vi "Cron Time to TimeStamp.vi"(10 "Correct for DST?":bool, 11 "Cron Time":T1) -> (3 "Time Stamp":timestamp)   [LabVIEW 2013, in "openCron.lvlib" / "Cron.lvclass"]
uses:
  Cron.lvclass
  CronTime -- cluster.ctl
  <vilib>/Utility/miscctls.llb/LVDateTimeRec.ctl
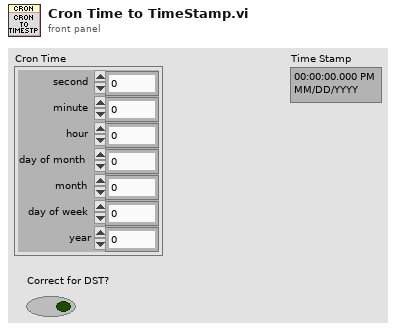
[diagram p1: front panel]
types:
  T1 = typedef "openCron.lvlib/Cron.lvclass/CronTime -- cluster.ctl" = cluster{"second":i32, "minute":i32, "hour":i32, "day of month":i32, "month":i32, "day of week":i32, "year":i32}
  T2 = typedef "LVDateTimeRec.ctl" = cluster{"fractional second":dbl, "second":i32, "minute":i32, "hour":i32, "day of month":i32, "month":i32, "year":i32, "day of week":i32, "day of year":i32, "DST":i32}
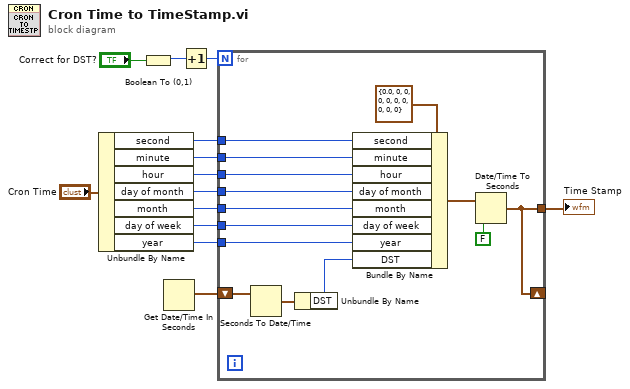
[diagram p0: block diagram]
diagram:
  n1 = Unbundle By Name("Cron Time") -> ("second"=w7:i32, "minute"=w8:i32, "hour"=w9:i32, "day of month"=w10:i32, "month"=w11:i32, "day of week"=w12:i32, "year"=w13:i32)
  n2 = Boolean To (0,1)(Boolean="Correct for DST?") -> (0, 1=w2:i16)
  n3 = Get Date/Time In Seconds() -> (seconds since 1Jan1904=w4:timestamp)
  n4 = Increment(x=w2) -> (x+1=w1:i16)
  n5 = for {
    N: w1 -> [_]
    tunnel: w13 -> [w27]
    tunnel: w12 -> [w26]
    tunnel: w11 -> [w25]
    tunnel: w10 -> [w24]
    tunnel: w9 -> [w23]
    tunnel: w8 -> [w22]
    tunnel: w7 -> [w21]
    tunnel: [w14] -> w5
    shift-right: [w14] -> _
    shift-left: w4 -> [w15]
    n6 = Seconds To Date/Time(time stamp (now)=w15) -> (date time rec=w17:T2)  [unwired: 1 in]
    n7 = Unbundle By Name(w17) -> ("DST"=w16:i32)
    n8 = Bundle By Name(cluster=T2 {"fractional second"=0.0, "second"=0, "minute"=0, "hour"=0, "day of month"=0, "month"=0, "year"=0, "day of week"=0, "day of year"=0, "DST"=0} ("date time rec"), "second"=w21, "minute"=w22, "hour"=w23, "day of month"=w24, "month"=w25, "day of week"=w26, "year"=w27, "DST"=w16) -> (w19:T2)
    n9 = Date/Time To Seconds(1:FALSE ("is UTC (F)"), 2:w19) -> (0:w14:timestamp)
  }
  "Time Stamp" <- w5
